vi "writeUART.vi"(8 "error in (no error)":errorcluster, 10 "write buffer":string, 11 "GiaoTiep in":refnum<class "GiaoTiepUART.lvclass">) -> (0 "error out":errorcluster, 2 "(DataWrite)":string, 3 "GiaoTiep out":refnum<class "GiaoTiepUART.lvclass">)   [LabVIEW 2014, in "LibraryGcode.lvlib" / "GiaoTiepUART.lvclass"]
uses:
  GiaoTiepUART.lvclass
  GiaoTiepUART.lvclass/GiaoTiepUART.ctl
  control/stateBoardFirmware.ctl
  LibraryGcode.lvlib
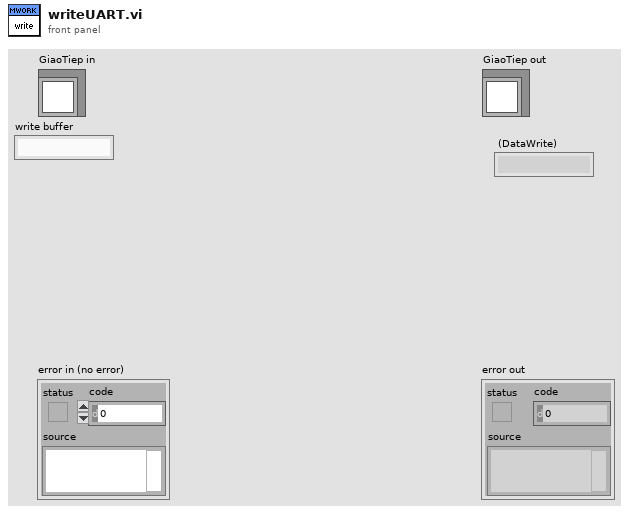
[diagram p1: front panel]
types:
  T1 = typedef "LibraryGcode.lvlib/stateBoardFirmware.ctl" = enum16{"Running", "Waiting", "Pos", "IDLE"}
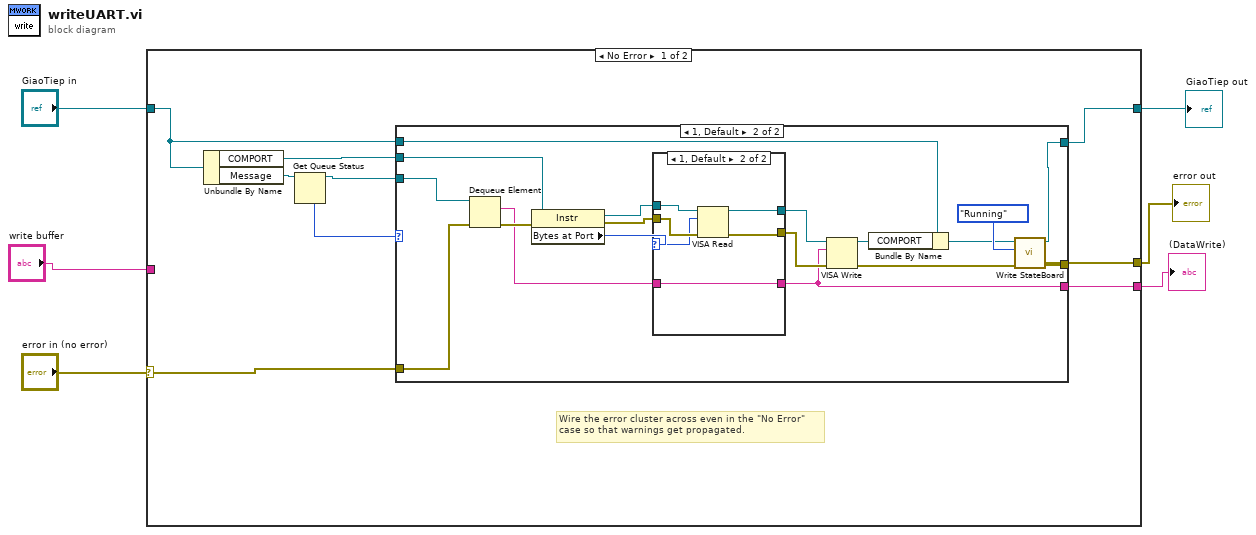
[diagram p0: block diagram]
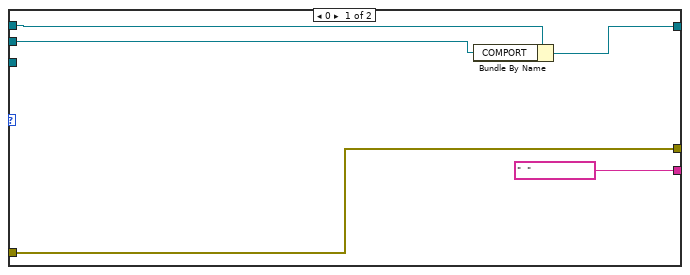
[diagram p2: hidden frame]
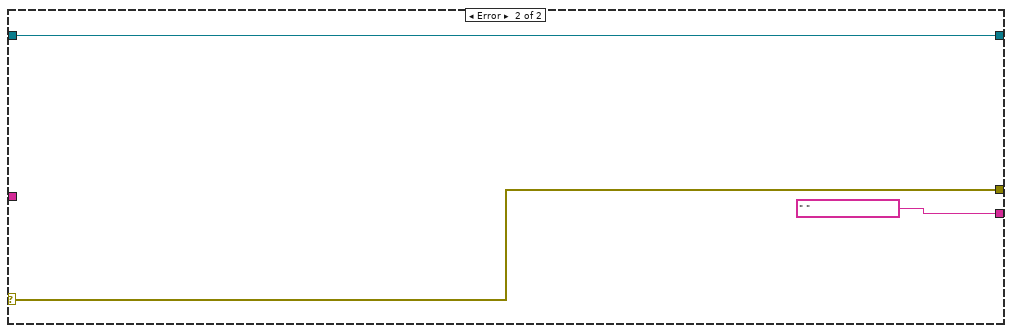
[diagram p4: hidden frame]
diagram:
  n1 = case shown="No Error" "error in (no error)" {
    selector: "error in (no error)" -> [w15 w50]
    tunnel: [w14 w50] -> w2
    tunnel: [w7 w49] -> w1
    tunnel: "GiaoTiep in" -> [w8 w49]
    tunnel: "write buffer" -> [_ _]
    tunnel: [w9 " " ("name (unnamed)")] -> w3
    frame No Error {
      # "Wire the error cluster across even in the \"No Error\"\ncase so that warnings get propagated."
      n2 = Unbundle By Name(w8) -> ("COMPORT"=w13:refnum<visa-resource-name>, "Message"=w12:refnum<queue>)
      n3 = Get Queue Status(queue=w12) -> (queue out=w10:refnum<queue>, # elements in queue=w11:i32)  [unwired: 2 in, 6 out]
      n4 = case shown="1, Default" w11 {
        tunnel: w15 -> [w20 w33]
        tunnel: [w20 w21] -> w14
        tunnel: w13 -> [w16 w34]
        tunnel: w10 -> [_ w31]
        tunnel: ["  " ("name (unnamed)") w29] -> w9
        tunnel: w8 -> [w18 w26]
        tunnel: [w17 w25] -> w7
        frame 0 {
          n5 = Bundle By Name(cluster=w18, "COMPORT"=w16) -> (w17:refnum<class "GiaoTiepUART.lvclass">)
        }
        frame 1, Default {
          n6 = Dequeue Element(queue=w31, error in (no error)=w33) -> (element=w30:string, error out=w32:errorcluster)  [unwired: 1 in, 2 out]
          n7 = property class="Instr"(reference=w34, error in=w32) -> (reference out=w38:refnum<visa-resource-name>, error out=w37:errorcluster, "Bytes at Port"=w22:u32)
          n8 = case shown="1, Default" w22 {
            selector: w22 -> [_ w45]
            tunnel: w38 -> [w41 w47]
            tunnel: w37 -> [w40 w46]
            tunnel: [w41 w43] -> w36
            tunnel: [w40 w42] -> w35
            tunnel: [w39 w44] -> w29
            tunnel: w30 -> [w39 w44]
            frame 0 {
            }
            frame 1, Default {
              n9 = VISA Read(VISA resource name=w47, byte count=w45, error in (no error)=w46) -> (VISA resource name out=w43:refnum<visa-resource-name>, error out=w42:errorcluster)  [unwired: 2 out]
            }
          }
          n10 = VISA Write(VISA resource name=w36, write buffer=w29, error in (no error)=w35) -> (VISA resource name out=w27:refnum<visa-resource-name>, error out=w28:errorcluster)  [unwired: 1 out]
          n11 = Bundle By Name(cluster=w26, "COMPORT"=w27) -> (w23:refnum<class "GiaoTiepUART.lvclass">)
          n12 = call-dynamic "Write StateBoard.vi"("error in (no error)"=w28, "StatePos"=stateBoardFirmware."Running", "XuLyStringUART in"=w23) -> ("error out"=w21:errorcluster, "XuLyStringUART out"=w25:refnum<class "GiaoTiepUART.lvclass">)  [unwired: 7 in]
        }
      }
    }
    frame Error {
    }
  }
  "error out" <- w2
  "GiaoTiep out" <- w1
  "(DataWrite)" <- w3
